vi "Untitled 2.vi"() -> ()   [LabVIEW 2017]
uses:
  Message Queue/Message Cluster.ctl
  Message Queue/Message Queue.lvlib
panel:
  out "HEX String 2":string
  out "HEX String":string
  out "data string":string
  out "Message Cluster 2":T1
  in  "Message Cluster":T1
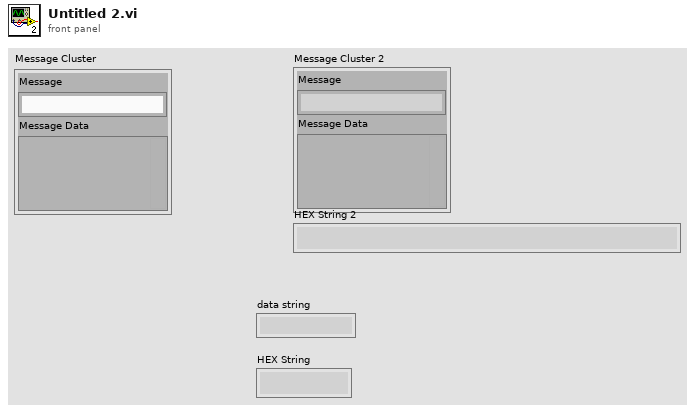
[diagram p1: front panel]
types:
  T1 = typedef "Message Queue.lvlib/Message Cluster.ctl" = cluster{"Message":string, "Message Data":variant}
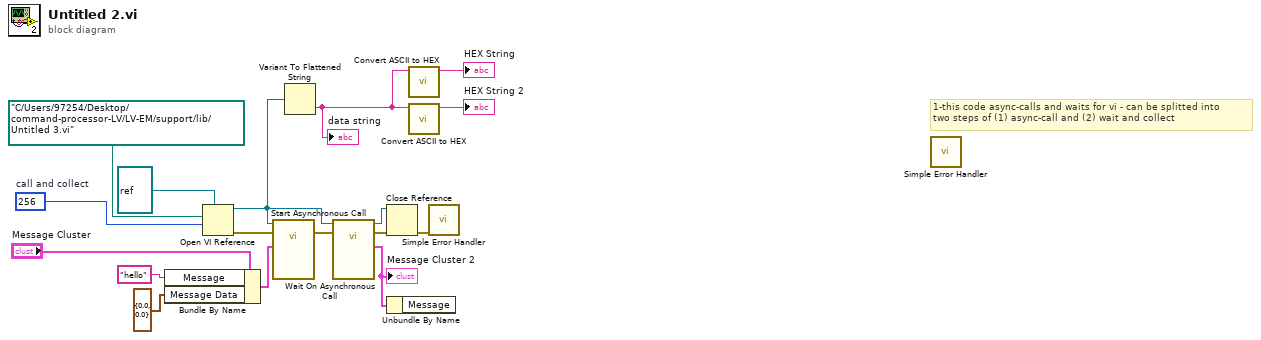
[diagram p0: block diagram]
diagram:
  w17 = 256  # call and collect
  # "1-this code async-calls and waits for vi - can be splitted into \ntwo steps of (1) async-call and (2) wait and collect"
  n1 = Bundle By Name(cluster="Message Cluster", "Message"="hello", "Message Data"=cluster{"X":dbl, "Y":dbl} {"X"=0.0, "Y"=0.0} ("output cluster")) -> (w9:T1)
  n2 = Open VI Reference(type specifier VI Refnum (for type only)=refnum<vi> refnum, vi path=path "C:/Users/97254/Desktop/command-processor-LV/LV-EM/support/lib/Untitled 3.vi", options=w17) -> (vi reference=w5:refnum<vi>, error out=w12:errorcluster)  [unwired: 3 in]
  n3 = call-by-ref "Start Asynchronous Call"(reference=w5, error in=w12, "Message Cluster"=w9) -> (error out=w1:errorcluster)  [unwired: 10 in, 2 out]
  n4 = Variant To Flattened String(Variant=w5) -> (data string=w3:string)  [unwired: 1 out]
  "data string" <- w3
  n5 = call-by-ref "Wait On Asynchronous Call"(reference=w5, error in=w1) -> (reference out=w14:refnum<vi>, error out=w13:errorcluster, "Message Cluster 2"=w8:T1)  [unwired: 11 in]
  "Message Cluster 2" <- w8
  n6 = Close Reference(reference=w14, error in (no error)=w13) -> (error out=w15:errorcluster)
  n7 = Unbundle By Name(w8) -> ()  [unwired: 1 out]
  n8 = call <userlib>:"Convert ASCII to HEX.vi"("ASCII String"=w3) -> ("HEX String"=→"HEX String":string)  [unwired: 10 in]
  n9 = call <userlib>:"Convert ASCII to HEX.vi"("ASCII String"=w3) -> ("HEX String"=→"HEX String 2":string)  [unwired: 10 in]
  n10 = call <vilib>:"Simple Error Handler.vi"("error in (no error)"=w15) -> ()  [unwired: 4 in, 5 out]
  n11 = call <vilib>:"Simple Error Handler.vi"() -> ()  [unwired: 5 in, 5 out]
